vi "TLCCS Identification Query.vi"(8 "error in (no error)":errorcluster {"code" format="%.0x"}, 11 "instrument handle":refnum<visa-resource-name>) -> (0 "error out":errorcluster {"code" format="%.0x"}, 1 "Device Name":string, 2 "Manufacturer Name":string, 3 "instrument handle out":refnum<visa-resource-name>, 4 "Serial Number":string, 5 "Firmware Revision":string, 6 "Instrument Driver Revision":string)   [LabVIEW 2020]
doc: "This VI returns the device identification information."
uses:
  tlccs_32.dll
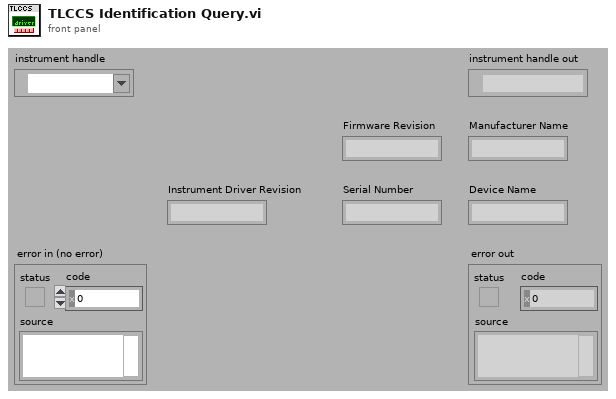
[diagram p1: front panel]
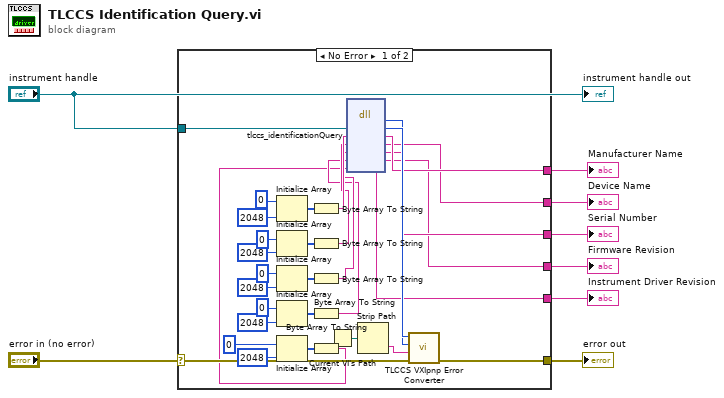
[diagram p0: block diagram]
diagram:
  n1 = case shown="No Error" "error in (no error)" {
    selector: "error in (no error)" -> [w35 w41]
    tunnel: [w34 w41] -> w8
    tunnel: "instrument handle" -> [w39 _]
    tunnel: [w29 _] -> w5
    tunnel: [w24 _] -> w4
    tunnel: [w19 _] -> w3
    tunnel: [w14 _] -> w2
    tunnel: [w9 _] -> w1
    frame No Error {
      n2 = Initialize Array(u8 0 ("element"), 2048 ("dimension size")) -> (w32:u8[])
      n3 = Initialize Array(u8 0 ("element"), 2048 ("dimension size")) -> (w27:u8[])
      n4 = Initialize Array(u8 0 ("element"), 2048 ("dimension size")) -> (w22:u8[])
      n5 = Initialize Array(u8 0 ("element"), 2048 ("dimension size")) -> (w17:u8[])
      n6 = Initialize Array(u8 0 ("element"), 2048 ("dimension size")) -> (w12:u8[])
      n7 = Byte Array To String(unsigned byte array=w32) -> (string=w33:string)
      n8 = Byte Array To String(unsigned byte array=w27) -> (string=w28:string)
      n9 = Byte Array To String(unsigned byte array=w22) -> (string=w23:string)
      n10 = Byte Array To String(unsigned byte array=w17) -> (string=w18:string)
      n11 = Byte Array To String(unsigned byte array=w12) -> (string=w13:string)
      n12 = Current VI's Path() -> (path=w40:path)
      n13 = dll-call lib="tlccs_32.*" fn="tlccs_identificationQuery"("Instrument Handle"=w39, "Manufacturer Name"=w33, "Device Name"=w28, "Serial Number"=w23, "Firmware Revision"=w18, "Instrument Driver Revision"=w13) -> (w37:i32, "Instrument Handle"=w38:u32, "Manufacturer Name"=w29:string, "Device Name"=w24:string, "Serial Number"=w19:string, "Firmware Revision"=w14:string, "Instrument Driver Revision"=w9:string)  [unwired: 3 in, 2 out]
      n14 = Strip Path(path=w40) -> (name=w36:string)  [unwired: 1 out]
      n15 = call "TLCCS VXIpnp Error Converter.vi"("error in (no error)"=w35, "name of VI (\"\")"=w36, "CVI error code (0)"=w37, "instrument handle"=w38) -> ("error out"=w34:errorcluster)  [unwired: 6 in, 1 out]
    }
    frame Error {
    }
  }
  "error out" <- w8
  "Manufacturer Name" <- w5
  "Device Name" <- w4
  "Serial Number" <- w3
  "Firmware Revision" <- w2
  "Instrument Driver Revision" <- w1
  "instrument handle out" <- "instrument handle"
